vi "controlActorSelection.vi"(7 "set":bool, 8 "error in":errorcluster, 9 "Positioner in":string, 10 "axis":u8(ring) items=["1", "2", "3"], 11 "connection ID":refnum<k5>) -> (0 "error out":errorcluster, 1 "Positioner out":string, 2 "axis out":u8, 3 "connection ID out":refnum<k5>, 4 "allPositioners":string[](array[string]))   [LabVIEW 2016, in "AMC_VIs.lvlib"]
doc: "With this VI the connected positioner type can be set or the currently in the system set positioner type can be read out (depending on the boolean input). In addition, a list of positioners can be retrieved, that can be set in the system."
uses:
  AMC_VIs.lvlib
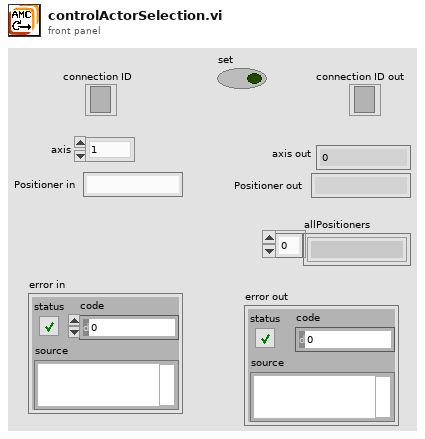
[diagram p1: front panel]
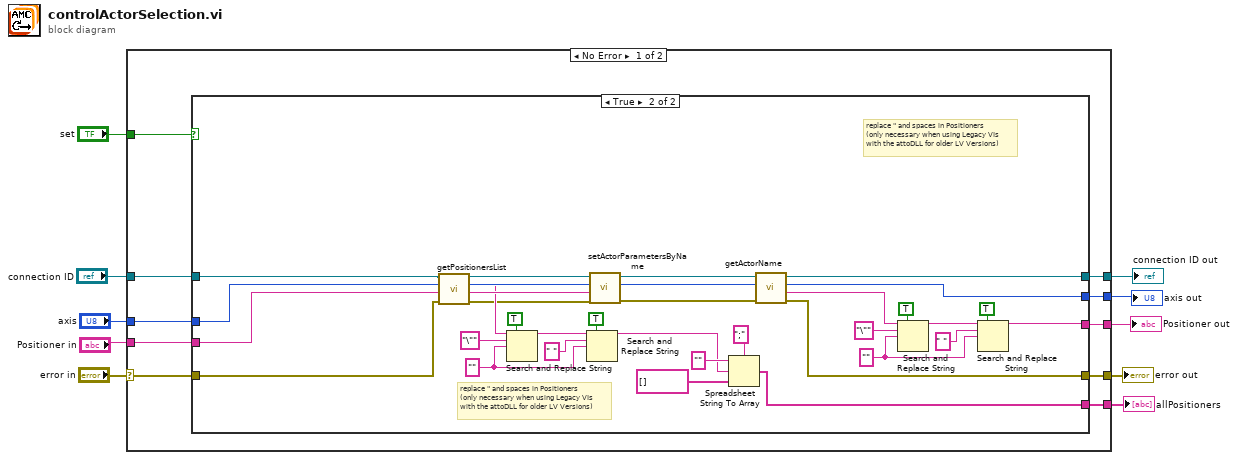
[diagram p0: block diagram]
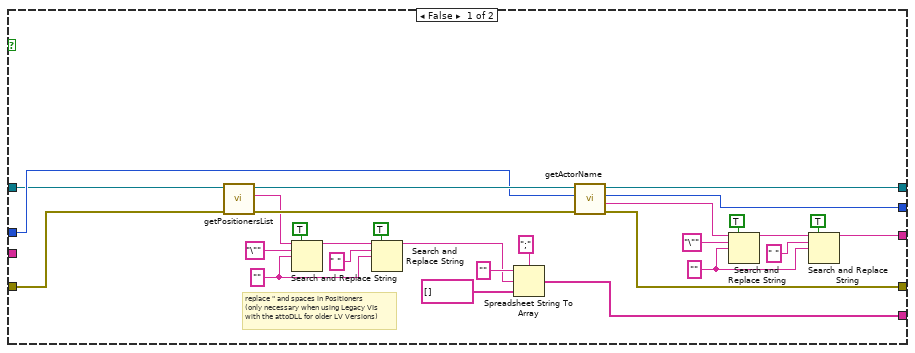
[diagram p2: hidden frame]
diagram:
  n1 = case shown="No Error" "error in" {
    selector: "error in" -> [w19 w83]
    tunnel: "axis" -> [w17 w84]
    tunnel: [w18 w83] -> w10
    tunnel: [w16 w84] -> w9
    tunnel: "Positioner in" -> [w15 w82]
    tunnel: [w20 w81] -> w2
    tunnel: "set" -> [w14 _]
    tunnel: [w13 w82] -> w5
    tunnel: [w12 _] -> w4
    tunnel: "connection ID" -> [w11 w81]
    frame No Error {
      n2 = case shown="True" w14 {
        tunnel: [w48 w77] -> w20
        tunnel: w19 -> [w40 w53]
        tunnel: [w46 w75] -> w18
        tunnel: w17 -> [w41 w80]
        tunnel: [w47 w73] -> w16
        tunnel: w15 -> [_ w79]
        tunnel: [w22 w65] -> w13
        tunnel: [w38 w51] -> w12
        tunnel: w11 -> [w21 w50]
        frame False {
          w26 = "" ("replace string (\"\")")
          w32 = "" ("replace string (\"\")")
          # "replace \" and spaces in Positioners\n(only necessary when using Legacy VIs\nwith the attoDLL for older LV Versions)"
          n3 = call "getPositionersList.vi"("error in"=w40, "connection ID"=w21) -> ("error out"=w39:errorcluster, "PositionersList"=w37:string, "connection ID"=w42:refnum<k5>)  [unwired: 7 in]
          n4 = Search and Replace String(replace all?=TRUE ("replace all? (F)"), input string=w37, search string="\"", replace string=w32) -> (result string=w36:string)  [unwired: 4 in, 3 out]
          n5 = Search and Replace String(replace all?=TRUE ("replace all? (F)"), input string=w36, search string=" ", replace string=w32) -> (result string=w35:string)  [unwired: 4 in, 3 out]
          n6 = Spreadsheet String To Array(delimiter (Tab)=";", format string="", spreadsheet string=w35, array type (2D Dbl)=string[] []) -> (array=w38:string[])
          n7 = call "getActorName.vi"("error in"=w39, "axis"=w41, "connection ID"=w42) -> ("error out"=w46:errorcluster, "actor_name"=w23:string, "axis_out"=w47:i32, "connection ID"=w48:refnum<k5>)  [unwired: 5 in]
          n8 = Search and Replace String(replace all?=TRUE ("replace all? (F)"), input string=w23, search string="\"", replace string=w26) -> (result string=w29:string)  [unwired: 4 in, 3 out]
          n9 = Search and Replace String(replace all?=TRUE ("replace all? (F)"), input string=w29, search string=" ", replace string=w26) -> (result string=w22:string)  [unwired: 4 in, 3 out]
        }
        frame True {
          w56 = "" ("replace string (\"\")")
          w69 = "" ("replace string (\"\")")
          # "replace \" and spaces in Positioners\n(only necessary when using Legacy VIs\nwith the attoDLL for older LV Versions)"
          # "replace \" and spaces in Positioners\n(only necessary when using Legacy VIs\nwith the attoDLL for older LV Versions)"
          n10 = call "getPositionersList.vi"("error in"=w53, "connection ID"=w50) -> ("error out"=w52:errorcluster, "PositionersList"=w61:string, "connection ID"=w49:refnum<k5>)  [unwired: 7 in]
          n11 = Search and Replace String(replace all?=TRUE ("replace all? (F)"), input string=w61, search string="\"", replace string=w56) -> (result string=w60:string)  [unwired: 4 in, 3 out]
          n12 = Search and Replace String(replace all?=TRUE ("replace all? (F)"), input string=w60, search string=" ", replace string=w56) -> (result string=w59:string)  [unwired: 4 in, 3 out]
          n13 = call "setActorParametersByName.vi"("error in"=w52, "actorname"=w79, "axis"=w80, "connection ID"=w49) -> ("error out"=w76:errorcluster, "axis_out"=w74:i32, "connection ID"=w78:refnum<k5>)  [unwired: 5 in]
          n14 = Spreadsheet String To Array(delimiter (Tab)=";", format string="", spreadsheet string=w59, array type (2D Dbl)=string[] []) -> (array=w51:string[])
          n15 = call "getActorName.vi"("error in"=w76, "axis"=w74, "connection ID"=w78) -> ("error out"=w75:errorcluster, "actor_name"=w66:string, "axis_out"=w73:i32, "connection ID"=w77:refnum<k5>)  [unwired: 5 in]
          n16 = Search and Replace String(replace all?=TRUE ("replace all? (F)"), input string=w66, search string="\"", replace string=w69) -> (result string=w72:string)  [unwired: 4 in, 3 out]
          n17 = Search and Replace String(replace all?=TRUE ("replace all? (F)"), input string=w72, search string=" ", replace string=w69) -> (result string=w65:string)  [unwired: 4 in, 3 out]
        }
      }
    }
    frame Error {
    }
  }
  "error out" <- w10
  "axis out" <- w9
  "Positioner out" <- w5
  "allPositioners" <- w4
  "connection ID out" <- w2
